vi "WireWriteBlockDiagram.vi"(8 "error in":errorcluster, 10 "Terminal References":T3, 11 "State":T1={"paths"={"index cluster path"=path "C:/Users/bcelis.AMER/Documents/TBDCore/source/Utilities/Cluster to Tag Bus Scripts/Controls/IndexCluster.ctl", "cluster path"=path "C:/Users/bcelis.AMER/Documents/TBDCore/source/Utilities/Cluster to Tag Bus Scripts/Controls/SampleControl.ctl", "cluster to tag bus VI path"=path "C:/Users/bcelis.AMER/Documents/TBDCore/source/Utilities/Cluster to Tag Bus Scripts/ClustertoTagbus.vi", " tag bus to cluster VI path"=path ""}, "write VI ref"=refnum, "read VI ref"=refnum, "base cluster"=variant}) -> (0 "error out":errorcluster, 3 "State out":T1={"paths"={"index cluster path"=path "C:/Users/bcelis.AMER/Documents/TBDCore/source/Utilities/Cluster to Tag Bus Scripts/Controls/IndexCluster.ctl", "cluster path"=path "C:/Users/bcelis.AMER/Documents/TBDCore/source/Utilities/Cluster to Tag Bus Scripts/Controls/SampleControl.ctl", "cluster to tag bus VI path"=path "C:/Users/bcelis.AMER/Documents/TBDCore/source/Utilities/Cluster to Tag Bus Scripts/ClustertoTagbus.vi", " tag bus to cluster VI path"=path ""}, "write VI ref"=refnum, "read VI ref"=refnum, "base cluster"=variant})   [LabVIEW 2013]
uses:
  Controls/TerminalReferences.ctl
  Controls/StateCluster.ctl
  Controls/PathsCluster.ctl
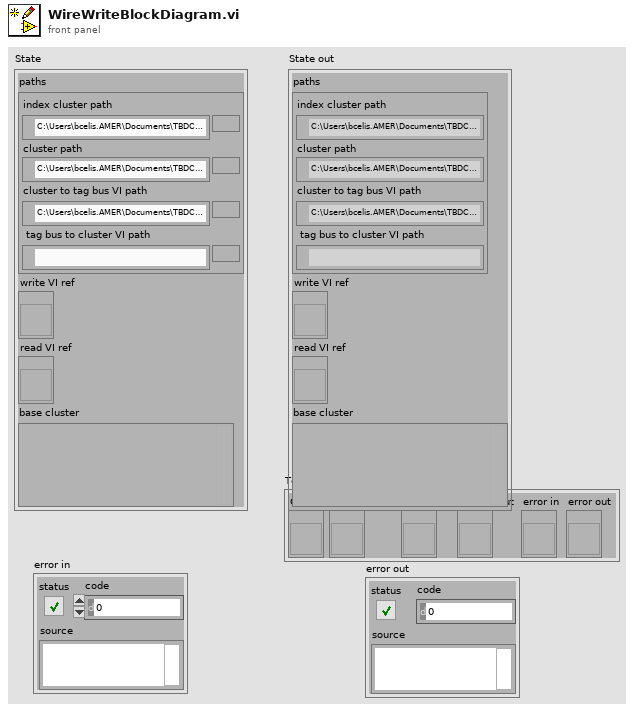
[diagram p1: front panel]
types:
  T1 = typedef "StateCluster.ctl" = cluster{"paths":T2, "write VI ref":refnum<vi>, "read VI ref":refnum<vi>, "base cluster":variant}
  T2 = typedef "PathsCluster.ctl" = cluster{"index cluster path":path, "cluster path":path, "cluster to tag bus VI path":path, " tag bus to cluster VI path":path}
  T3 = typedef "TerminalReferences.ctl" = cluster{"Cluster":refnum<vi>, "Index Cluster":refnum<vi>, "tag bus in":refnum<vi>, "tag bus out":refnum<vi>, "error in ":refnum<vi>, "error out":refnum<vi>}
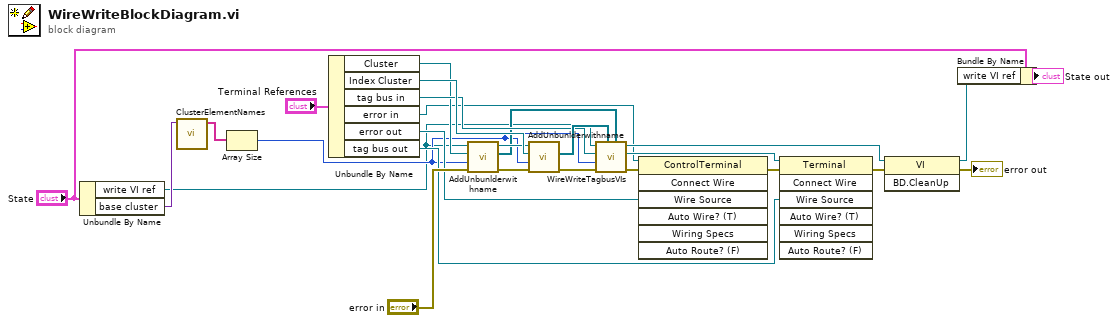
[diagram p0: block diagram]
diagram:
  n1 = Unbundle By Name("State") -> ("write VI ref"=w1:refnum<vi>, "base cluster"=w22:variant)
  n2 = call "ClusterElementNames.vi"("input cluster"=w22) -> ("Elements Names"=w21:string[])  [unwired: 8 in, 2 out]
  n3 = Array Size(array=w21) -> (size(s)=w2:i32)
  n4 = Unbundle By Name("Terminal References") -> ("Cluster"=w15:refnum<vi>, "Index Cluster"=w24:refnum<vi>, "tag bus in"=w17:refnum<vi>, "error in"=w6:refnum<vi>, "error out"=w8:refnum<vi>, "tag bus out"=w7:refnum<vi>)
  n5 = call "AddUnbunlderwithname.vi"("error in"="error in", "elements in cluster"=w2, "cluster terminal"=w15, "VI in"=w1) -> ("error out"=w13:errorcluster, "terminals"=w3:refnum<vi>[], "VI out"=w14:refnum<vi>)  [unwired: 5 in]
  n6 = call "AddUnbunlderwithname.vi"("error in"=w13, "elements in cluster"=w2, "cluster terminal"=w24, "VI in"=w14) -> ("error out"=w5:errorcluster, "terminals"=w23:refnum<vi>[])  [unwired: 5 in, 1 out]
  n7 = call "WireWriteTagbusVIs.vi"("terminals data"=w3, "terminals indexes"=w23, "error in"=w5, "elements in cluster"=w2, "tag bus in in"=w17, "VI in"=w1) -> ("error out"=w4:errorcluster, "tag bus out"=w9:refnum<vi>, "VI out"=w12:refnum<vi>)  [unwired: 3 in]
  n8 = invoke on="Invoke Node" class="ControlTerminal" method="Connect Wire"(reference=w6, error in=w4, "Wire Source"=w8) -> (error out=w11:errorcluster)  [unwired: 4 in, 6 out]
  n9 = invoke on="Invoke Node" class="Terminal" method="Connect Wire"(reference=w9, error in=w11, "Wire Source"=w7) -> (error out=w10:errorcluster)  [unwired: 4 in, 6 out]
  n10 = invoke class="VI" method="BD.CleanUp"(reference=w12, error in=w10) -> (reference out=w18:refnum<vi>, error out=→"error out":errorcluster)  [unwired: 1 in, 1 out]
  n11 = Bundle By Name(cluster="State", "write VI ref"=w18) -> (→"State out":T1)
